vi "Close Handle.vi"(0 "instrument handle":refnum<k15>[](array[refnum]), 2 "Software Flags":T1, 11 "error in (no error)":errorcluster) -> (15 "error out":errorcluster)   [LabVIEW 2024, in "devicePowerSequencerCoreLogic.lvlib"]
uses:
  devicePowerSequencerCoreLogic.lvlib
  controls/Software Flags.ctl
  Common/Error Message.vi
  <vilib>/Utility/error.llb/Error Cluster From Error Code.vi
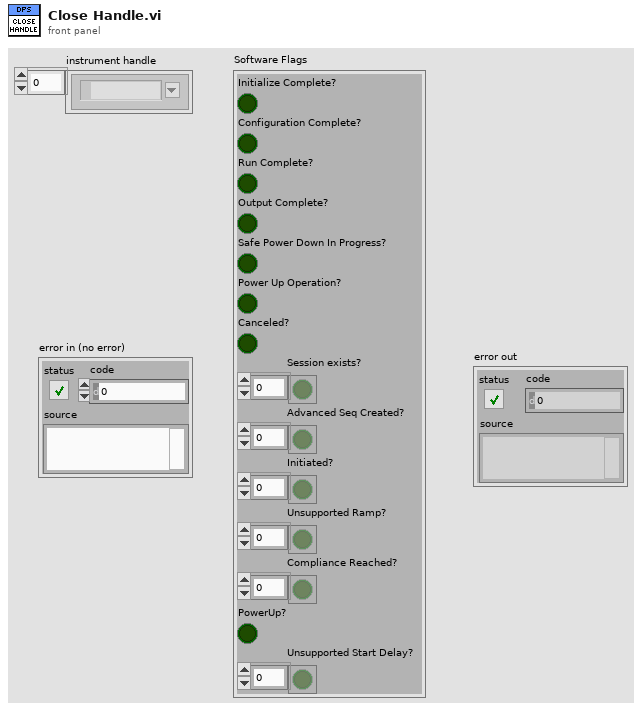
[diagram p1: front panel]
types:
  T1 = typedef "devicePowerSequencerCoreLogic.lvlib/Software Flags.ctl" = cluster{"Initialize Complete?":bool, "Configuration Complete?":bool, "Run Complete?":bool, "Output Complete?":bool, "Safe Power Down In Progress?":bool, "Power Up Operation?":bool, "Canceled?":bool, "Session exists?":bool[], "Advanced Seq Created?":bool[], "Initiated?":bool[], "Unsupported Ramp?":bool[], "Compliance Reached?":bool[], "PowerUp?":bool, "Unsupported Start Delay?":bool[]}
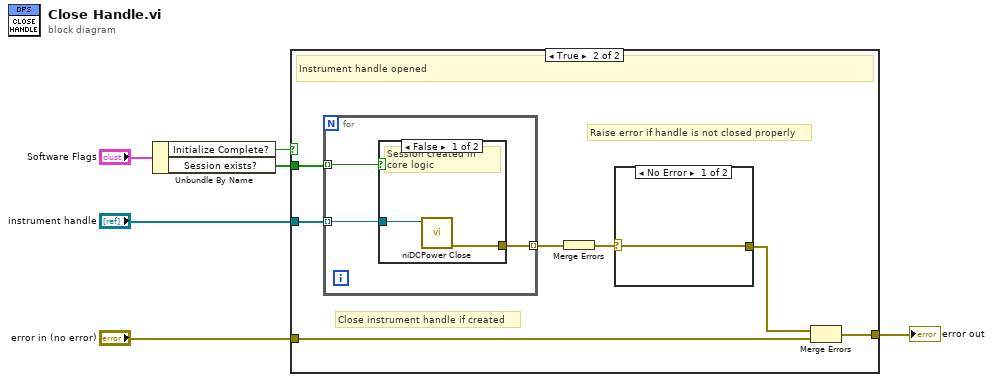
[diagram p0: block diagram]
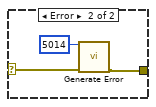
[diagram p3: hidden frame]
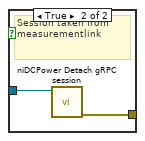
[diagram p4: hidden frame]
diagram:
  n1 = Unbundle By Name("Software Flags") -> ("Initialize Complete?"=w2:bool, "Session exists?"=w1:bool[])
  n2 = case shown="True" w2 {
    tunnel: "error in (no error)" -> [w7 w11]
    tunnel: "instrument handle" -> [_ w12]
    tunnel: [w7 w13] -> w4
    tunnel: w1 -> [_ w14]
    frame False {
      # "Instrument Handle not opened"
    }
    frame True {
      # "Raise error if handle is not closed properly"
      # "Close instrument handle if created"
      # "Instrument handle opened"
      n3 = for {
        tunnel: w12 -> [w21] mode=indexing
        tunnel: w14 -> [w19] mode=indexing
        tunnel: [w20] -> w10 mode=indexing
        n4 = case shown="False" w19 {
          tunnel: w21 -> [w23 w25]
          tunnel: [w22 w24] -> w20
          frame False {
            # "Session created in core logic"
            n5 = call <instrlib>:"niDCPower Close.vi"("instrument handle"=w23) -> ("error out"=w22:errorcluster)  [unwired: 10 in]
          }
          frame True {
            # "Session taken from measurementlink"
            n6 = call <instrlib>:"niDCPower Detach gRPC session.vi"("instrument handle"=w25) -> ("error out"=w24:errorcluster)  [unwired: 10 in]
          }
        }
      }
      n7 = Merge Errors(w10) -> (w8:errorcluster)
      n8 = case shown="No Error" w8 {
        selector: w8 -> [w15 w18]
        tunnel: [w15 w16] -> w9
        frame No Error {
        }
        frame Error {
          n9 = call "Generate Error.vi"("Error Code"=5014, "error in (no error)"=w18) -> ("error out"=w16:errorcluster)  [unwired: 13 in]
        }
      }
      n10 = Merge Errors(w9, w11) -> (w13:errorcluster)
    }
  }
  "error out" <- w4
